vi "_save_csv_ENA_Recorder.vi"(5 "Marker_array":dbl[](array[numeric]), 7 "NoteName":string="SingleCh_", 11 "array in":string[][](array[string])) -> (3 "FileName":string)   [LabVIEW 2023]
uses:
  <vilib>/Utility/file.llb/Write Delimited Spreadsheet (string).vi
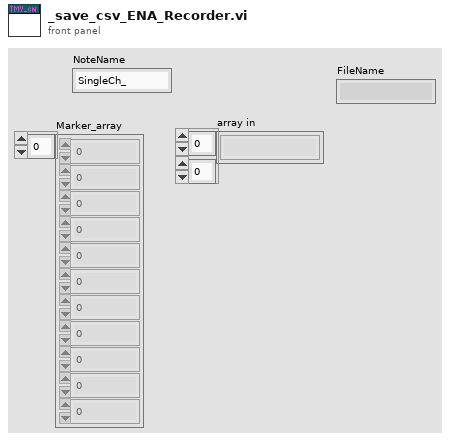
[diagram p1: front panel]
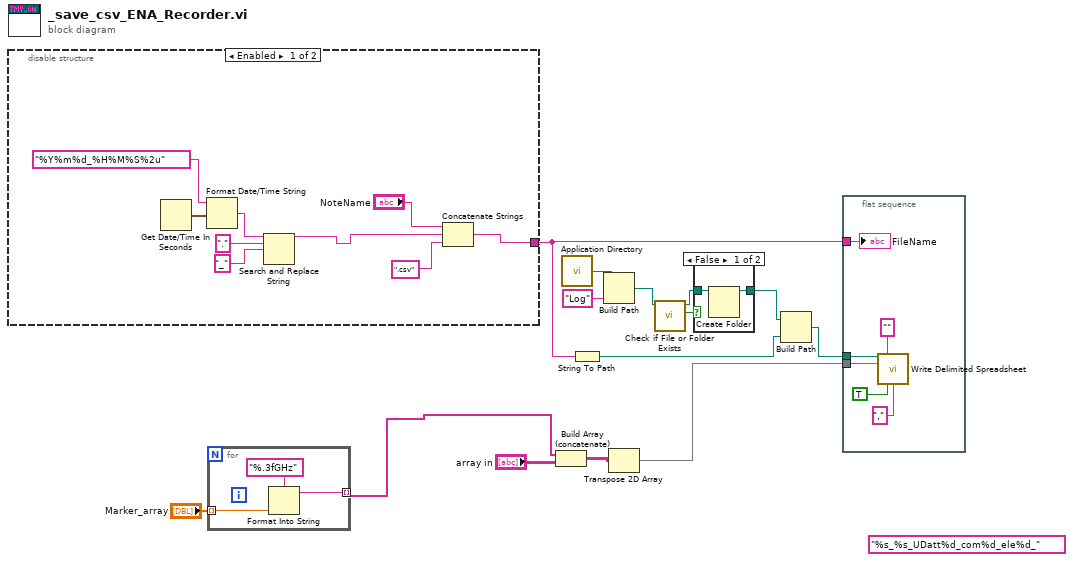
[diagram p0: block diagram]
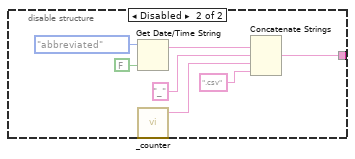
[diagram p3: hidden frame]
diagram:
  (unwired) "%s_%s_UDatt%d_com%d_ele%d_" ("format string")
  n1 = disable-structure shown="Enabled" {
    disable-tunnel: [w22 w24] -> w11
    frame Enabled {
      n2 = Get Date/Time In Seconds() -> (seconds since 1Jan1904=w20:timestamp)
      n3 = Format Date/Time String(time format string (%c)="%Y%m%d_%H%M%S%2u", seconds (now)=w20) -> (date/time string=w18:string)  [unwired: 1 in]
      n4 = Search and Replace String(input string=w18, search string=".", replace string="_") -> (result string=w15:string)  [unwired: 5 in, 3 out]
      n5 = Concatenate Strings("NoteName", w15, ".csv" ("delimiter (\\t)")) -> (w22:string)
    }
    frame Disabled {
      n6 = Get Date/Time String(date format (0)=enum16{"short", "long", "abbreviated"}."abbreviated", want seconds? (F)=FALSE) -> (date string=w31:string)  [unwired: 1 in, 1 out]
      n7 = call "_counter.vi"() -> ("out_count"=w25:string)  [unwired: 5 in]
      n8 = Concatenate Strings(w31, "_" ("delimiter (\\t)"), w25, ".csv" ("delimiter (\\t)")) -> (w24:string, w26:string)
    }
  }
  n9 = for {
    tunnel: "Marker_array" -> [w34] mode=indexing
    tunnel: [w32] -> w1 mode=indexing
    n10 = Format Into String(format string="%.3fGHz", w34) -> (resulting string=w32:string)  [unwired: 2 in, 1 out]
  }
  n11 = Build Array (concatenate)(w1, "array in") -> (w3:string[][])
  n12 = call <vilib>:"Application Directory.vi"() -> ("Application Directory"=w10:path)
  n13 = String To Path(string=w11) -> (path=w13:path)
  n14 = Build Path(base path=w10, name or relative path="Log") -> (appended path=w7:path)
  n15 = Transpose 2D Array(2D array=w3) -> (transposed array=w5:string[][])
  n16 = call <vilib>:"Check if File or Folder Exists.vi"("path"=w7) -> ("file or folder exists?"=w9:bool, "dup path"=w8:path)  [unwired: 8 in, 1 out]
  n17 = case shown="False" w9 {
    tunnel: w8 -> [w36 w37]
    tunnel: [w35 w37] -> w6
    frame False {
      n18 = Create Folder(path (use dialog)=w36) -> (created path=w35:path)  [unwired: 2 in, 2 out]
    }
    frame True {
    }
  }
  n19 = Build Path(base path=w6, name or relative path=w13) -> (appended path=w12:path)
  n20 = flat-sequence {
    tunnel: w12 -> [w42]
    tunnel: w11 -> [w40]
    tunnel: w5 -> [w38]
    frame #0 {
      n21 = call-poly <vilib>:"Write Delimited Spreadsheet.vi"("file path (dialog if empty)"=w42, "format (%s)"="" ("format (%.3f)"), "2D data"=w38, "transpose? (no:F)"=TRUE, "delimiter (\\t)"="," ("delimiter (\\t)")) -> ()  [unwired: 9 in, 2 out]
      "FileName" <- w40
    }
  }
